vi "WPI_DashboardLog NetworkTables2.vi"(6 "Robot IP":string, 8 "UDP Control":string, 9 "TCP":string, 10 "UDP Status":string, 11 "NT Data Values":T5(array[cluster])) -> ()   [LabVIEW 2017]
uses:
  <vilib>/Rock Robotics/Network Tables/Protocol Operations.ctl
  <vilib>/Rock Robotics/Network Tables/Field Data.ctl
  <vilib>/Rock Robotics/Network Tables/Field Type.ctl
  <vilib>/Rock Robotics/Network Tables/Sequence.ctl
  <vilib>/Rock Robotics/Network Tables/Make Table Operation.ctl
  <vilib>/Rock Robotics/WPI/Dashboard/WPI_DashboardLoggingRecord.ctl
  <vilib>/Rock Robotics/WPI/Dashboard/WPI_DashboardNTL Header Type.ctl
  <vilib>/Rock Robotics/WPI/Dashboard/WPI_DashboardLogging Global.vi
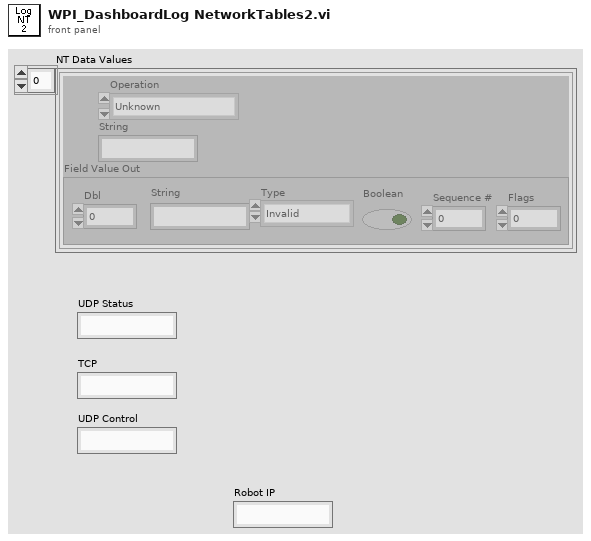
[diagram p1: front panel]
types:
  T1 = typedef "Protocol Operations.ctl" = enum16{"Unknown", "Keep Alive", "Client Hello", "Version not supported", "Server Hello Complete", "Assign", "Update", "No Op", "Server Hello", "Client Hello Complete", "Update Flags", "Delete Entry", "Delete All", "RPC Exec", "RPC Response"}
  T2 = typedef "Field Data.ctl" = cluster{"Dbl":dbl, "String":string, "Type":T3, "Boolean":bool, "Sequence #":T4, "Flags":u8}
  T3 = typedef "Field Type.ctl" = enum8{"Invalid", "Bool", "Numeric", "String", "Raw", "Boolean Array", "Numeric Array", "String Array", "RPC"}
  T4 = typedef "Sequence.ctl" = u16
  T5 = cluster{"Operation":T1, "String":string, "Field Value Out":T2}[]
  T6 = typedef "WPI_DashboardNTL Header Type.ctl" = cluster{"Version":i32, "Duration (ms)":i32, "TimeStamp":timestamp, "Robot IP":string, "Displays":string[]}
  T7 = typedef "WPI_DashboardLoggingRecord.ctl" = cluster{"time Ofst":i32, "video index":i32, "video index 2":i32, "video index 3":i32, "video index 4":i32, "UDP Status":string, "TCP":string, "UDP Control":string, "NT Updates":cluster{"Operation":T1, "Name":string, "Field Value":T2}[]}
  T8 = typedef "Make Table Operation.ctl" = enum16{"Get or Add Field", "Get Field or Add Temp", "Replace Temp ID", "Get Field ID - No Add", "Get Table Field IDs", "Get Field ID Info", "Move Field to Temp", "Validate", "Remove Field", "Remove All"}
  T9 = enum16{"open", "replace", "create", "open or create", "replace or create", "replace or create with confirmation"}
  T10 = cluster{"Operation":T1, "Name":string, "Field Value":T2}[]
  T11 = cluster{"Video 1":i32, "Video 2":i32, "Video 3":i32, "Video 4":i32}
  T12 = typedef "Field ID.ctl" = i32
  T13 = cluster{"Operation":T1, "String":string, "Field Value Out":T2}
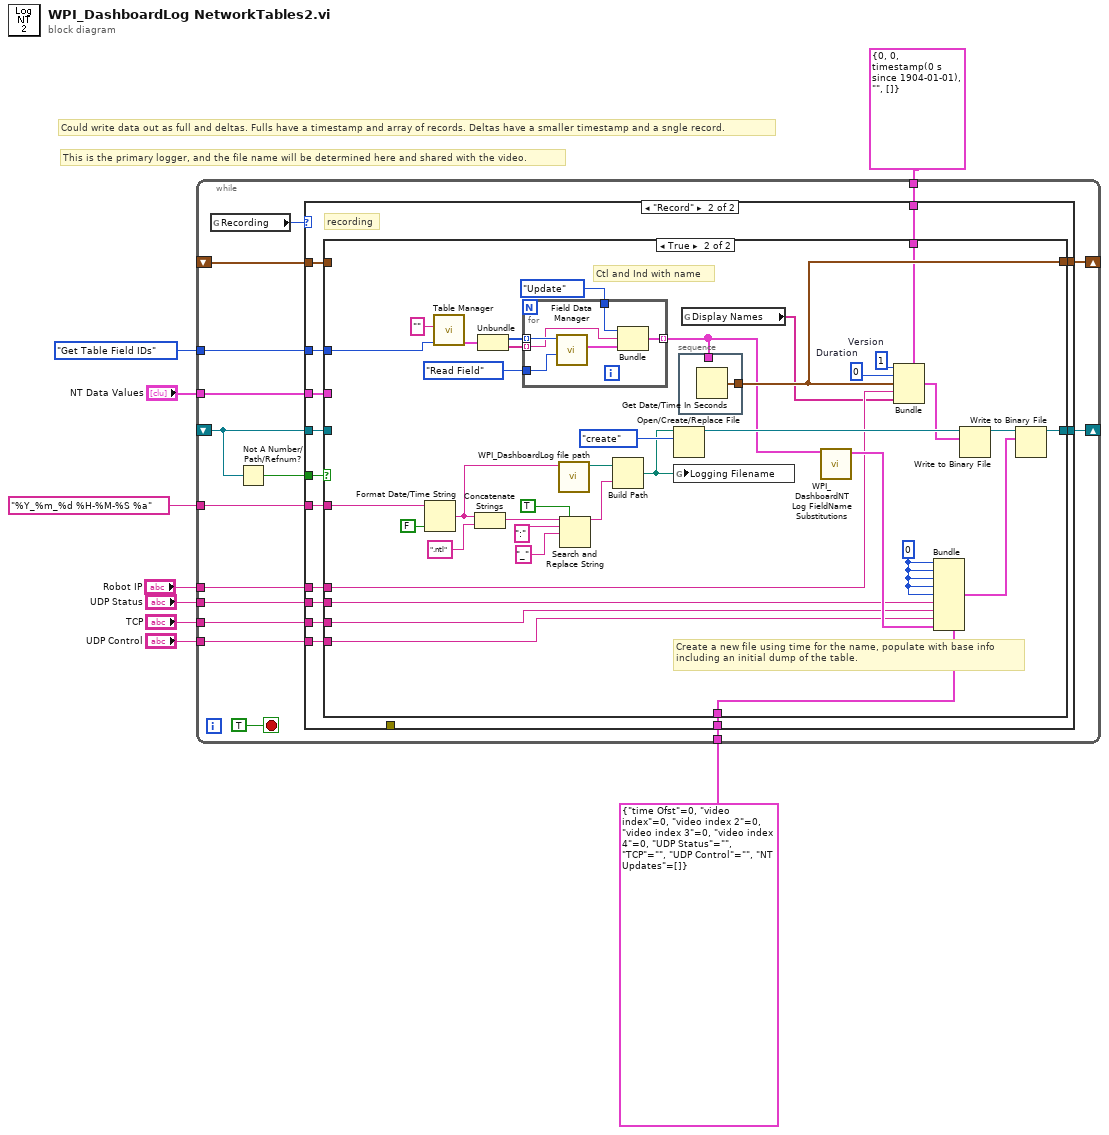
[diagram p0: block diagram]
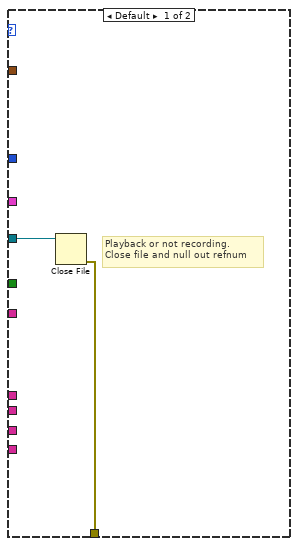
[diagram p2: hidden frame]
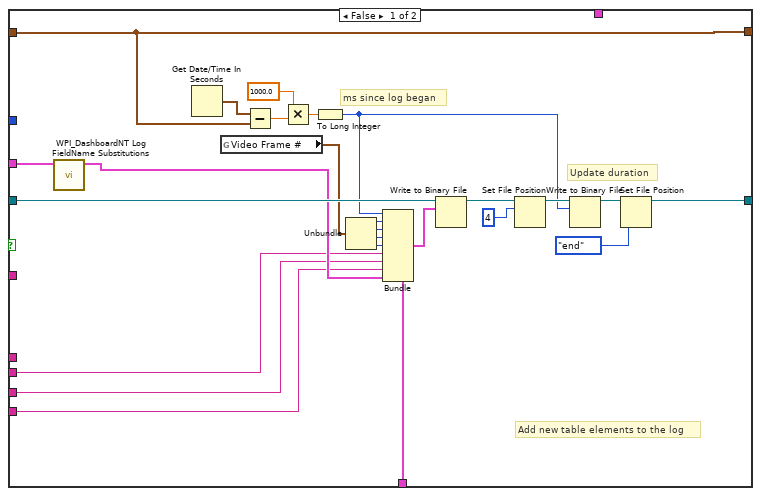
[diagram p3: hidden frame]
diagram:
  # "Could write data out as full and deltas. Fulls have a timestamp and array of records. Deltas have a smaller timestamp and a sngle record."
  # "This is the primary logger, and the file name will be determined here and shared with the video."
  n1 = while {
    shift-right: [w24] -> _
    shift-left: _ -> [w21]
    tunnel: Make_Table_Operation."Get Table Field IDs" ("Operation") -> [w23]
    tunnel: "NT Data Values" -> [w22]
    tunnel: "%Y_%m_%d %H-%M-%S %a" ("time format string (%c)") -> [w18]
    shift-right: [w17] -> _
    shift-left: _ -> [w16]
    tunnel: T7 {"time Ofst"=0, "video index"=0, "video index 2"=0, "video index 3"=0, "video index 4"=0, "UDP Status"="", "TCP"="", "UDP Control"="", "NT Updates"=[]} ("output cluster") -> [w15]
    tunnel: "UDP Status" -> [w14]
    tunnel: "TCP" -> [w13]
    tunnel: "UDP Control" -> [w12]
    tunnel: "Robot IP" -> [w11]
    tunnel: T6 {"Version"=0, "Duration (ms)"=0, "TimeStamp"=timestamp(0 s since 1904-01-01), "Robot IP"="", "Displays"=[]} ("Header") -> [w10]
    stop <- TRUE stop-if-true
    n2 = global read "WPI_DashboardLogging Global.vi" "Recording"() -> (w19:enum32{"Stop", "Record", "Playback"})
    n3 = Not A Number/Path/Refnum?(number/path/refnum=w21) -> (NaN/Path/Refnum?=w20:bool)
    n4 = case shown="\"Record\"" w19 {
      tunnel: [_ w41] -> w24
      tunnel: w23 -> [_ w40]
      tunnel: w22 -> [_ w39]
      tunnel: w21 -> [w26 w38]
      tunnel: w20 -> [_ w37]
      tunnel: w18 -> [_ w36]
      tunnel: [_ w35] -> w17
      tunnel: w16 -> [_ w34]
      tunnel: [w27 _] -> _
      tunnel: w15 -> [_ w33]
      tunnel: w14 -> [_ w32]
      tunnel: w13 -> [_ w31]
      tunnel: w12 -> [_ w30]
      tunnel: w11 -> [_ w29]
      tunnel: w10 -> [_ w28]
      frame Default {
        # "Playback or not recording.\nClose file and null out refnum"
        n5 = Close File(refnum=w26) -> (error out=w27:errorcluster)  [unwired: 1 in, 1 out]
      }
      frame "Record" {
        # "recording"
        n6 = case shown="True" w37 {
          tunnel: [w64 w82] -> w41
          tunnel: w40 -> [_ w93]
          tunnel: w38 -> [w66 _]
          tunnel: w39 -> [w54 _]
          tunnel: w36 -> [_ w90]
          tunnel: [w65 w81] -> w35
          tunnel: w34 -> [w65 _]
          tunnel: w33 -> [w53 w77]
          tunnel: w32 -> [w50 w74]
          tunnel: w31 -> [w49 w73]
          tunnel: w30 -> [w48 w72]
          tunnel: w29 -> [_ w71]
          tunnel: w28 -> [_ w68]
          frame False {
            # "Update duration"
            # "ms since log began"
            # "Add new table elements to the log"
            n7 = call <vilib>:"WPI_DashboardNT Log FieldName Substitutions.vi"("Updates in"=w54) -> ("Updates out"=w51:T10)  [unwired: 10 in]
            n8 = Get Date/Time In Seconds() -> (seconds since 1Jan1904=w63:timestamp)
            n9 = global read "WPI_DashboardLogging Global.vi" "Video Frame #"() -> (w46:T11)
            n10 = Subtract(x=w63, y=w65) -> (x-y=w62:dbl)
            n11 = Multiply(x=1000.0, y=w62) -> (x*y=w61:dbl)
            n12 = To Long Integer(number=w61) -> (32bit integer=w47:i32)
            n13 = Unbundle(w46) -> ("Video 1"=w45:i32, "Video 2"=w44:i32, "Video 3"=w43:i32, "Video 4"=w42:i32)
            n14 = Bundle(cluster=w53, "time Ofst"=w47, "video index"=w45, "video index 2"=w44, "video index 3"=w43, "video index 4"=w42, "UDP Status"=w50, "TCP"=w49, "UDP Control"=w48, "NT Updates"=w51) -> (w52:T7)
            n15 = Write to Binary File(file (use dialog)=w66, data=w52) -> (refnum out=w57:refnum<file>)  [unwired: 4 in, 2 out]
            n16 = Set File Position(offset (in bytes) (0)=i64 4, refnum=w57) -> (refnum out=w56:refnum<file>)  [unwired: 2 in, 1 out]
            n17 = Write to Binary File(file (use dialog)=w56, data=w47) -> (refnum out=w59:refnum<file>)  [unwired: 4 in, 2 out]
            n18 = Set File Position(refnum=w59, from (0:start)=enum16{"start", "end", "current"}."end") -> (refnum out=w64:refnum<file>)  [unwired: 2 in, 1 out]
          }
          frame True {
            w70 = 0
            w79 = 0  # Duration
            w80 = 1  # Version
            # "Create a new file using time for the name, populate with base info\nincluding an initial dump of the table."
            # "Ctl and Ind with name"
            n19 = Format Date/Time String(time format string (%c)=w90, UTC format=FALSE) -> (date/time string=w69:string)  [unwired: 1 in]
            n20 = call <vilib>:"Table Manager.vi"("Operation"=w93, "Entry Name"="") -> ("Entries"=w101:cluster{"Entry IDs":T12[], "Names":string[]})  [unwired: 6 in, 3 out]
            n21 = Concatenate Strings(w69, ".ntl" ("time format string (%c)")) -> (w85:string)
            n22 = Unbundle(w101) -> ("Entry IDs"=w102:T12[], "Names"=w103:string[])
            n23 = for {
              tunnel: w102 -> [w109] mode=indexing
              tunnel: [w108] -> w78 mode=indexing
              tunnel: enum16{"Update Field", "Read Field"}."Read Field" ("Operation") -> [w110]
              tunnel: w103 -> [w107] mode=indexing
              tunnel: Protocol_Operations."Update" ("Operation") -> [w105]
              n24 = call <vilib>:"Field Data Manager.vi"("Operation"=w110, "Field ID"=w109) -> ("Field Value Out"=w106:T2)  [unwired: 8 in, 1 out]
              n25 = Bundle("Operation"=w105, "String"=w107, "Field Value Out"=w106) -> (w108:T13)  [unwired: 1 in]
            }
            n26 = call <vilib>:"WPI_DashboardLog file path.vi"("Time Date String"=w69) -> ("appended path"=w98:path)  [unwired: 10 in]
            n27 = Search and Replace String(replace all?=TRUE ("replace all? (F)"), input string=w85, search string=":", replace string="_") -> (result string=w84:string)  [unwired: 4 in, 3 out]
            n28 = Build Path(base path=w98, name or relative path=w84) -> (appended path=w92:path)
            n29 = Open/Create/Replace File(file path (use dialog)=w92, operation (0:open)=T9."create") -> (refnum out=w95:refnum<file>)  [unwired: 4 in, 2 out]
            n30 = global write "WPI_DashboardLogging Global.vi" "Logging Filename"(w92) -> ()
            n31 = stacked-sequence {
              tunnel: [w104] -> w81
              tunnel: w78 -> [_]
              frame #0 {
                n32 = Get Date/Time In Seconds() -> (seconds since 1Jan1904=w104:timestamp)
              }
            }
            n33 = global read "WPI_DashboardLogging Global.vi" "Display Names"() -> (w67:string[])
            n34 = call <vilib>:"WPI_DashboardNT Log FieldName Substitutions.vi"("Updates in"=w78) -> ("Updates out"=w76:T10)  [unwired: 10 in]
            n35 = Bundle(cluster=w68, "Version"=w80, "Duration (ms)"=w79, "TimeStamp"=w81, "Robot IP"=w71, "Displays"=w67) -> (w94:T6)
            n36 = Bundle(cluster=w77, "time Ofst"=w70, "video index"=w70, "video index 2"=w70, "video index 3"=w70, "video index 4"=w70, "UDP Status"=w74, "TCP"=w73, "UDP Control"=w72, "NT Updates"=w76) -> (w75:T7)
            n37 = Write to Binary File(file (use dialog)=w95, data=w94) -> (refnum out=w83:refnum<file>)  [unwired: 4 in, 2 out]
            n38 = Write to Binary File(file (use dialog)=w83, data=w75) -> (refnum out=w82:refnum<file>)  [unwired: 4 in, 2 out]
          }
        }
      }
    }
  }
